vi "demo_zigzag.vi"() -> ()   [LabVIEW 2017]
panel:
  in  "step":dbl
  in  "Z+":bool
  in  "Z-":bool
  in  "X-":bool
  in  "X+":bool
  in  "Y-":bool
  in  "Y+":bool
  in  "origin to":bool
  in  "to":bool
  in  "n":i32=1
  in  "z":dbl
  in  "步进":bool
  out "posz":dbl
  out "pos y":dbl
  out "pos x":dbl
  in  "回零":bool
  in  "下一步":bool
  in  "v":dbl=10.0
  in  "y":dbl
  in  "x":dbl
  in  "停止":bool
  in  "确定按钮":bool
  in  "String":string(combo)="home"
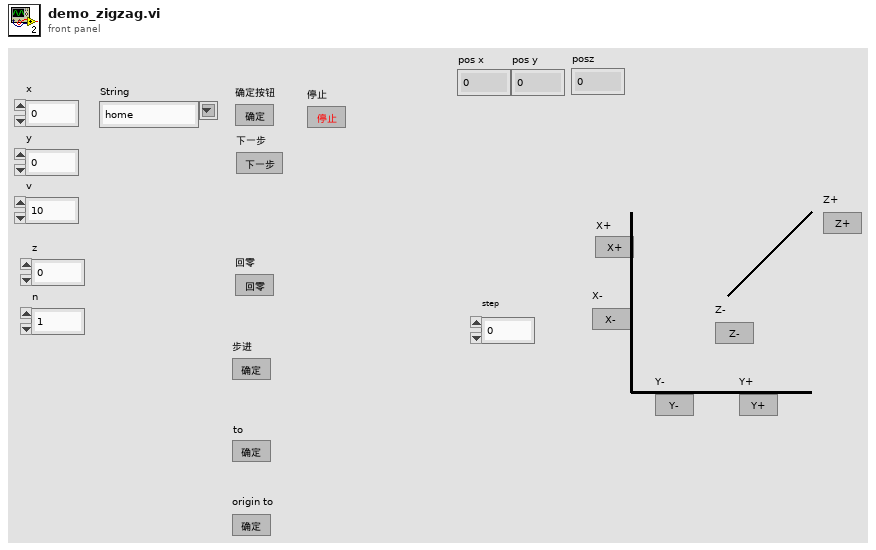
[diagram p1: front panel]
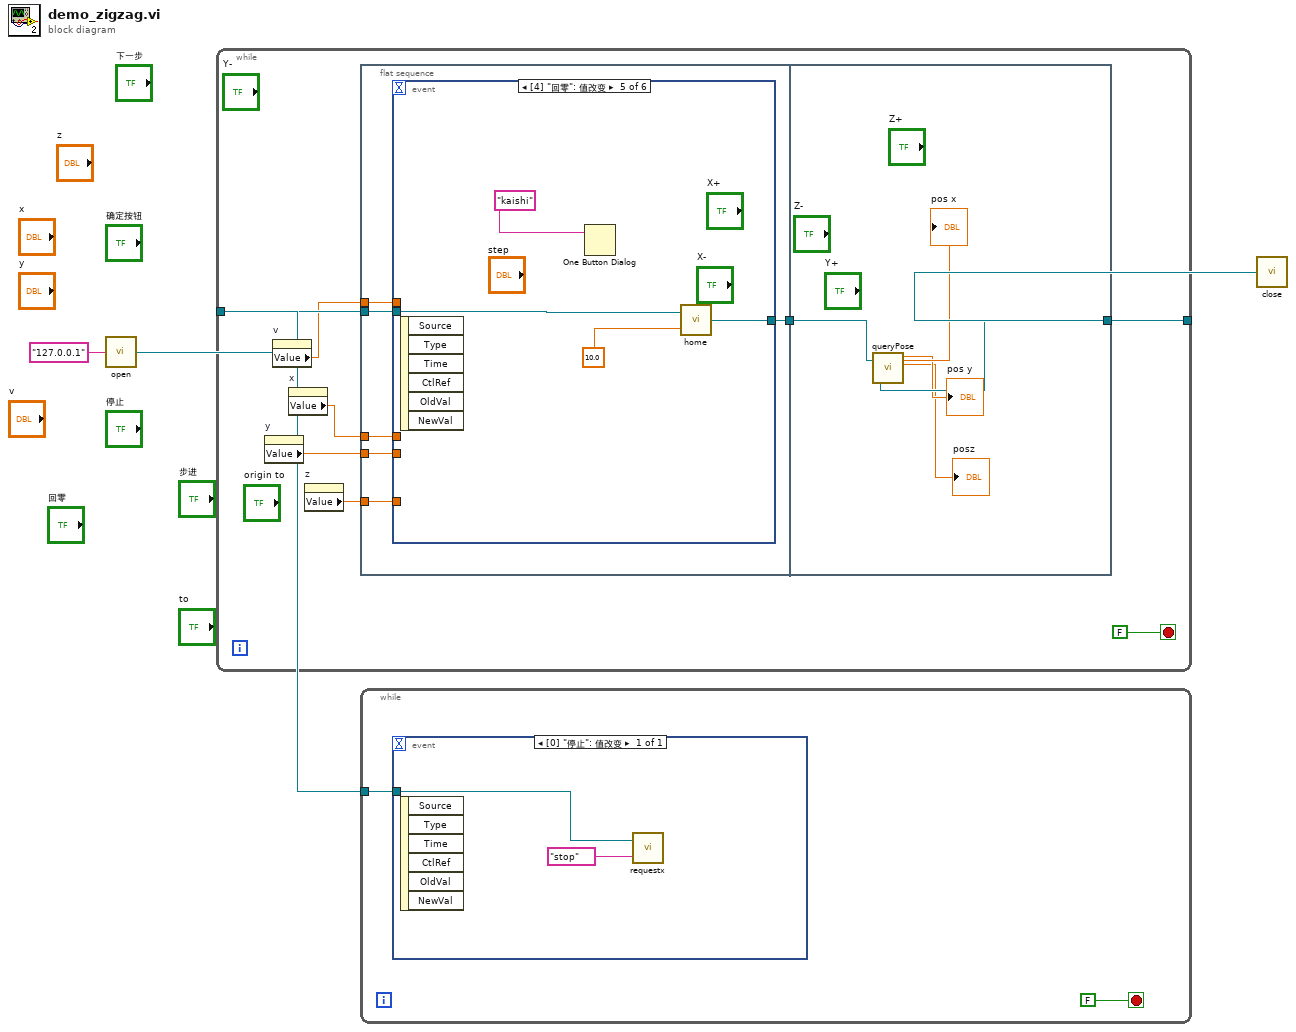
[diagram p0: block diagram]
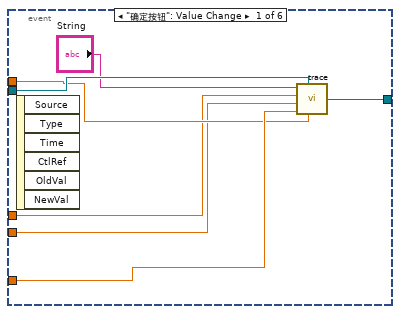
[diagram p2: hidden frame]
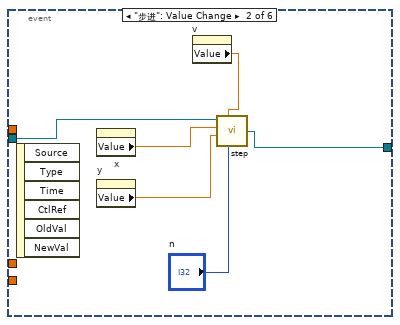
[diagram p3: hidden frame]
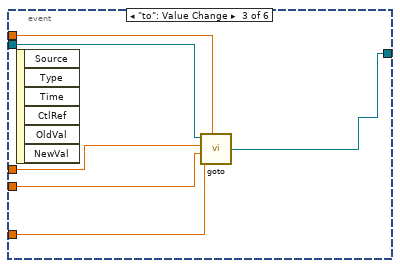
[diagram p4: hidden frame]
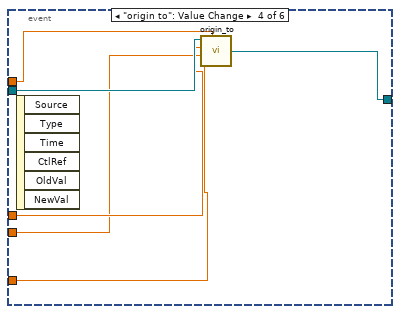
[diagram p5: hidden frame]
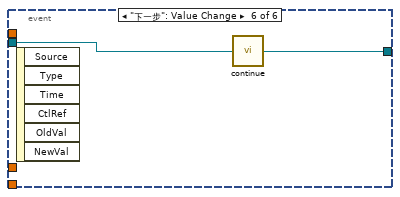
[diagram p6: hidden frame]
diagram:
  n1 = call "open.vi"("地址"="127.0.0.1") -> ("连接ID"=w2:refnum<k5>)
  n2 = while {
    tunnel: [w11] -> w3
    tunnel: w2 -> [w10]
    stop <- FALSE stop-if-true
    n3 = property on="y" class="DigNum (严格)"() -> ("Value"=w6:dbl)  [unwired: 2 in, 2 out]
    n4 = property on="v" class="DigNum (严格)"() -> ("Value"=w4:dbl)  [unwired: 2 in, 2 out]
    n5 = property on="x" class="DigNum (严格)"() -> ("Value"=w7:dbl)  [unwired: 2 in, 2 out]
    n6 = property on="z" class="DigNum (严格)"() -> ("Value"=w5:dbl)  [unwired: 2 in, 2 out]
    n7 = flat-sequence {
      tunnel: w10 -> [w16]
      tunnel: [w17] -> w8
      tunnel: w7 -> [w15]
      tunnel: w6 -> [w14]
      tunnel: w5 -> [w13]
      tunnel: w4 -> [w12]
      tunnel: [w52] -> w11
      tunnel: w8 -> [w53]
      frame #0 {
        n8 = event shown="[4] \"回零\": 值改变" {
          selector: _ -> [_ _ _ _ _ _]
          dyn-events: _ -> [_ _ _ _ _ _]
          timeout: _ -> [_ _ _ _ _ _]
          tunnel: [w24 w26 w35 w37 w44 w48] -> w17
          tunnel: w16 -> [w23 w27 w36 w42 w46 w47]
          tunnel: w15 -> [w19 _ w34 w40 _ _]
          tunnel: w14 -> [w18 _ w33 w39 _ _]
          tunnel: w13 -> [w21 _ w32 w38 _ _]
          tunnel: w12 -> [w20 _ w31 w41 _ _]
          event "确定按钮": Value Change {
            n9 = event-data() -> ()  [unwired: 1 in, 6 out]
            n10 = call "trace.vi"("v"=w20, "连接ID"=w23, "z"=w21, "y"=w18, "x"=w19, "type"="String") -> ("连接ID输出"=w24:refnum<k5>)
          }
          event "步进": Value Change {
            n11 = event-data() -> ()  [unwired: 1 in, 6 out]
            n12 = property on="x" class="DigNum (严格)"() -> ("Value"=w30:dbl)  [unwired: 2 in, 2 out]
            n13 = property on="y" class="DigNum (严格)"() -> ("Value"=w29:dbl)  [unwired: 2 in, 2 out]
            n14 = property on="v" class="DigNum (严格)"() -> ("Value"=w28:dbl)  [unwired: 2 in, 2 out]
            n15 = call "step.vi"("n"="n", "v"=w28, "y"=w29, "x"=w30, "连接ID"=w27) -> ("连接ID 2"=w26:refnum<k5>)  [unwired: 1 in]
          }
          event "to": Value Change {
            n16 = event-data() -> ()  [unwired: 1 in, 6 out]
            n17 = call "goto.vi"("连接ID"=w36, "x"=w34, "y"=w33, "z"=w32, "v"=w31) -> ("连接ID 2"=w35:refnum<k5>)
          }
          event "origin to": Value Change {
            n18 = event-data() -> ()  [unwired: 1 in, 6 out]
            n19 = call "origin_to.vi"("连接ID"=w42, "x"=w40, "y"=w39, "z"=w38, "v"=w41) -> ("连接ID 2"=w37:refnum<k5>)
          }
          event "回零": Value Change {
            n20 = event-data() -> ()  [unwired: 1 in, 6 out]
            n21 = One Button Dialog(message="kaishi" ("消息")) -> ()  [unwired: 1 in, 1 out]
            n22 = call "home.vi"("velocity"=10.0, "连接ID"=w46) -> ("连接ID 2"=w44:refnum<k5>)
          }
          event "下一步": Value Change {
            n23 = event-data() -> ()  [unwired: 1 in, 6 out]
            n24 = call "continue.vi"("连接ID"=w47) -> ("连接ID 2"=w48:refnum<k5>)
          }
        }
      }
      frame #1 {
        n25 = call "queryPose.vi"("连接ID"=w53) -> ("连接ID输出"=w52:refnum<k5>, "x"=→"pos x":dbl, "y"=→"pos y":dbl, "z"=→"posz":dbl)  [unwired: 3 out]
      }
    }
  }
  n26 = while {
    tunnel: w2 -> [w55]
    stop <- FALSE stop-if-true
    n27 = event shown="[0] \"停止\": 值改变" {
      selector: _ -> [_]
      dyn-events: _ -> [_]
      timeout: _ -> [_]
      tunnel: w55 -> [w56]
      event "停止": Value Change {
        n28 = event-data() -> ()  [unwired: 1 in, 6 out]
        n29 = call "requestx.vi"("cmd"="stop" ("String"), "连接ID"=w56) -> ()  [unwired: 1 out]
      }
    }
  }
  n30 = call "close.vi"("连接ID"=w3) -> ()
